vi "FT2232_V5.vi"(4 "ADC set":T1={"LED Selection"=enum."LED 6", "LED Power"=0}, 6 "BriLED set":T3={"LED Selection"=enum."Test 1 (POTW1)", "LED Power"=0}, 7 "LED selection":enum16{"FluLED", "BriLED", "ADCDAC"}(ring), 8 "error in":errorcluster, 9 "FulLED set":T3={"LED Selection"=enum."Test 1 (POTW1)", "LED Power"=0}, 10 "ADC_Channel":u32, 11 "LED event":T4(ring)) -> (0 "error out":errorcluster, 1 "Close result":i32=1, 2 "Initialize":T2, 3 "ADC_Data":u32)   [LabVIEW 2019, in "LED.lvlib"]
uses:
  LED.lvlib
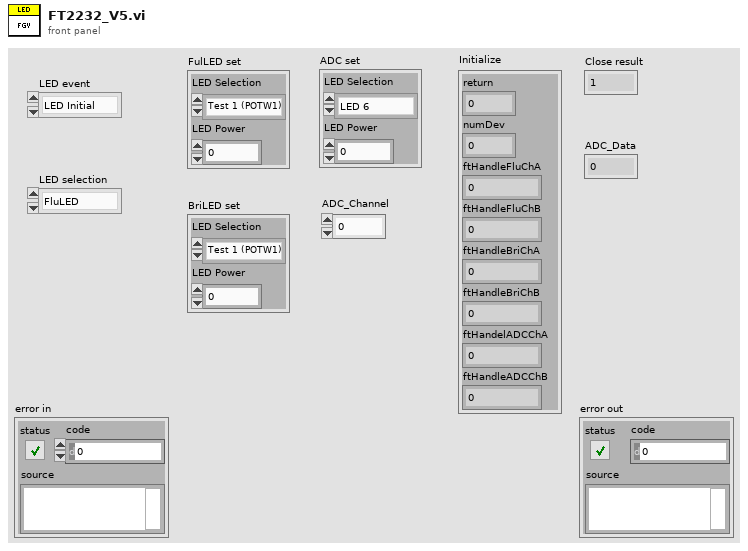
[diagram p1: front panel]
types:
  T1 = cluster{"LED Selection":enum8{"LED 1", "LED 2", "LED 3", "LED 4", "LED 5", "LED 6", "Test 1 (POTW1)"}, "LED Power":u8}
  T2 = cluster{"return":i32, "numDev":u32, "ftHandleFluChA":u32, "ftHandleFluChB":u32, "ftHandleBriChA":u32, "ftHandleBriChB":u32, "ftHandelADCChA":u32, "ftHandleADCChB":u32}
  T3 = cluster{"LED Selection":enum8{"LED 1", "LED 2", "LED 3", "LED 4", "LED 5", "Test 1 (POTW1)"}, "LED Power":u8}
  T4 = enum16{"LED Initial", "LED On", "LED Off", "LED Change", "LED Close", "ADC Read"}
  T5 = enum8{"LED 1", "LED 2", "LED 3", "LED 4", "LED 5", "Test 1 (POTW1)"}
  T6 = enum8{"LED 1", "LED 2", "LED 3", "LED 4", "LED 5", "LED 6", "Test 1 (POTW1)"}
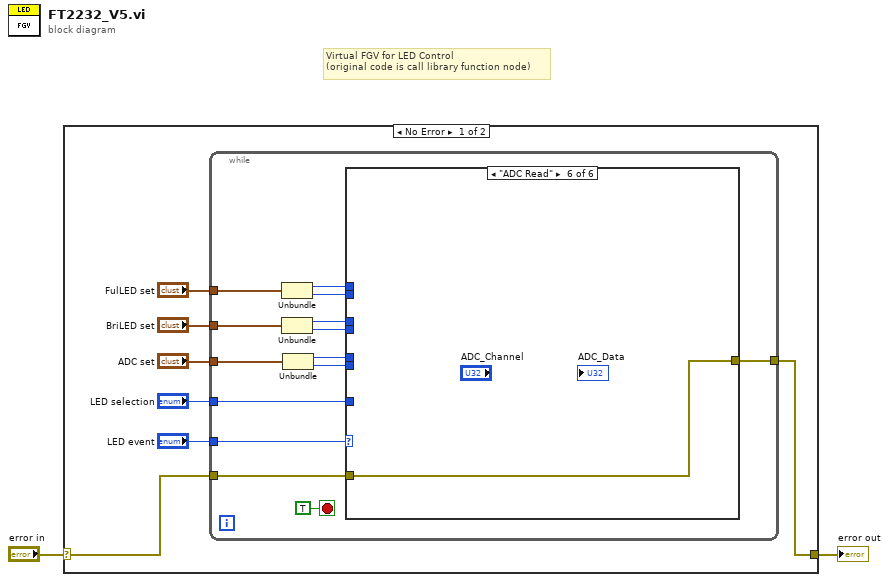
[diagram p0: block diagram]
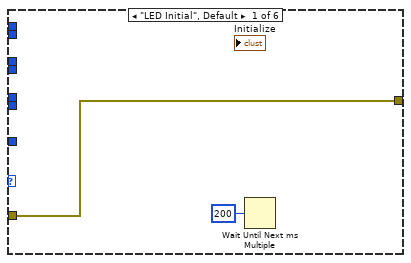
[diagram p2: hidden frame]
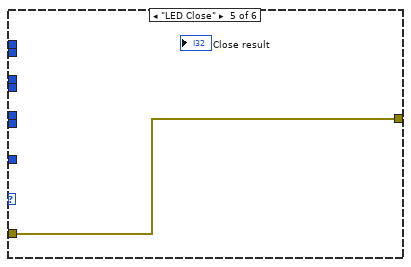
[diagram p12: hidden frame]
diagram:
  # "Virtual FGV for LED Control\n(original code is call library function node)"
  n1 = case shown="No Error" "error in" {
    selector: "error in" -> [w4 w58]
    tunnel: [w3 w58] -> w1
    frame No Error {
      n2 = while {
        tunnel: "LED event" -> [w22]
        tunnel: "LED selection" -> [w21]
        tunnel: "BriLED set" -> [w20]
        tunnel: "FulLED set" -> [w18]
        tunnel: "ADC set" -> [w14]
        tunnel: w4 -> [w11]
        tunnel: [w10] -> w3
        stop <- TRUE stop-if-true
        n3 = Unbundle(w18) -> ("LED Selection"=w17:T5, "LED Power"=w16:u8)
        n4 = Unbundle(w20) -> ("LED Selection"=w19:T5, "LED Power"=w15:u8)
        n5 = Unbundle(w14) -> ("LED Selection"=w13:T6, "LED Power"=w12:u8)
        n6 = case shown="\"ADC Read\"" w22 {
          tunnel: w21 -> [_ w31 w40 w52 _ _]
          tunnel: w19 -> [_ w30 w39 w51 _ _]
          tunnel: w17 -> [_ w29 w38 w49 _ _]
          tunnel: w16 -> [_ _ _ w48 _ _]
          tunnel: w15 -> [_ _ _ w50 _ _]
          tunnel: w13 -> [_ w28 w37 w47 _ _]
          tunnel: w12 -> [_ _ _ w46 _ _]
          tunnel: w11 -> [w24 w27 w36 w45 w56 w57]
          tunnel: [w24 w26 w35 w44 w56 w57] -> w10
          frame "LED Initial", Default {
            n7 = Wait Until Next ms Multiple(millisecond multiple=u32 200) -> ()  [unwired: 1 out]
          }
          frame "LED On" {
            n8 = case shown="\"BriLED\"" w31 {
              tunnel: w30 -> [_ _ _]
              tunnel: w29 -> [_ _ _]
              tunnel: w28 -> [_ _ _]
              tunnel: w27 -> [w32 w33 w34]
              tunnel: [w32 w33 w34] -> w26
              frame "FluLED", Default {
              }
              frame "BriLED" {
              }
              frame "ADCDAC" {
              }
            }
          }
          frame "LED Off" {
            n9 = case shown="\"FluLED\", Default" w40 {
              tunnel: w39 -> [_ _ _]
              tunnel: w38 -> [_ _ _]
              tunnel: w37 -> [_ _ _]
              tunnel: w36 -> [w41 w42 w43]
              tunnel: [w41 w42 w43] -> w35
              frame "FluLED", Default {
              }
              frame "BriLED" {
              }
              frame "ADCDAC" {
              }
            }
          }
          frame "LED Change" {
            n10 = case shown="\"BriLED\"" w52 {
              tunnel: w51 -> [_ _ _]
              tunnel: w50 -> [_ _ _]
              tunnel: w49 -> [_ _ _]
              tunnel: w48 -> [_ _ _]
              tunnel: w47 -> [_ _ _]
              tunnel: w46 -> [_ _ _]
              tunnel: w45 -> [w53 w54 w55]
              tunnel: [w53 w54 w55] -> w44
              frame "FluLED", Default {
              }
              frame "BriLED" {
              }
              frame "ADCDAC" {
              }
            }
          }
          frame "LED Close" {
          }
          frame "ADC Read" {
          }
        }
      }
    }
    frame Error {
    }
  }
  "error out" <- w1
